vi "PQC_VisualAlignment_contact.vi"() -> ()   [LabVIEW 2020]
uses:
  <vilib>/userdefined/High Color/IMAQdx.ctl
  <vilib>/vision/driver/IMAQdx.llb/IMAQdx Buffer Number Mode.ctl
  <vilib>/Analysis/baseanly.llb/Mean (DBL).vi
  <vilib>/Utility/file.llb/Read Delimited Spreadsheet (string).vi
  <instrlib>/Keithley 700B Series/Keithley 700B Series.lvlib
  <instrlib>/Agilent E4980/Agilent E4980.lvlib
  <vilib>/vision/driver/NI_Vision_Acquisition_Software.lvlib
  <vilib>/Analysis/NI_AALBase.lvlib
panel:
  in  "array 2":dbl[][](array[numeric])=[[999999999.0, 1000000000.0, 1000000000.0, 1000000000.0], [1000000000.0, 1000000000.0, 1000000000.0, 1000000000.0], [1000000000.0, 1000000000.0, 1000000000.0, 1000000000.0], [1000000000.0, 1000000000.0, 1000000000.0, 1000000000.0], [1000000000.0, 1000000000.0, 1000000000.0, 1000000000.0], [1000000000.0, 1000000000.0, 1000000000.0, 1000000000.0], [1000000000.0, 1000000000.0, 1000000000.0, 1000000000.0], [1000000000.0, 1000000000.0, 1000000000.0, 1000000000.0], [1000000000.0, 1000000000.0, 1000000000.0, 1000000000.0], [1000000000.0, 1000000000.0, 1000000000.0, 1000000000.0]] format="%_3e"
  in  "Switch Channel File Path":path=path "C:/Users/Lab User/Desktop/PQC_VisualAlignment/contactSwitchChannels.txt"
  in  "?":enum32{"Data", "Debug and Errors"}(tab)
  out "Rp":dbl[unit]
  out "Cp":dbl[unit]
  in  "Resistance Check":bool
  in  "Measurement Number":i32
  out "Measurement Set":i32
  out "Indicator Cluster":T1
  out "Average of last 3 measurements":dbl[](array[numeric])
  out "Error Out":errorcluster
  in  "stop camera":bool
  in  "Camera ID 2":T2="PQC top"
  out "Frame Rate":dbl
  in  "Start Camera":bool
  in  "Stop Program":bool
  in  "LCR VISA Resource":refnum<visa-resource-name>="GPIB0::19::INSTR"
  in  "707B VISA Resource":refnum<visa-resource-name>="GPIB0::16::INSTR"
  out "PQC Alignment":T3(plugin-control)
  # "2H11, 2B01, 1B01, 2B11, 2B03, 2B04, 2B05, 2B06, 2B07, 2B08, 1H02, 1H03, 1H04, 1H05, 1H06, 1H07, 1H08, 1H09, 2H09, 2H02, 1A11"
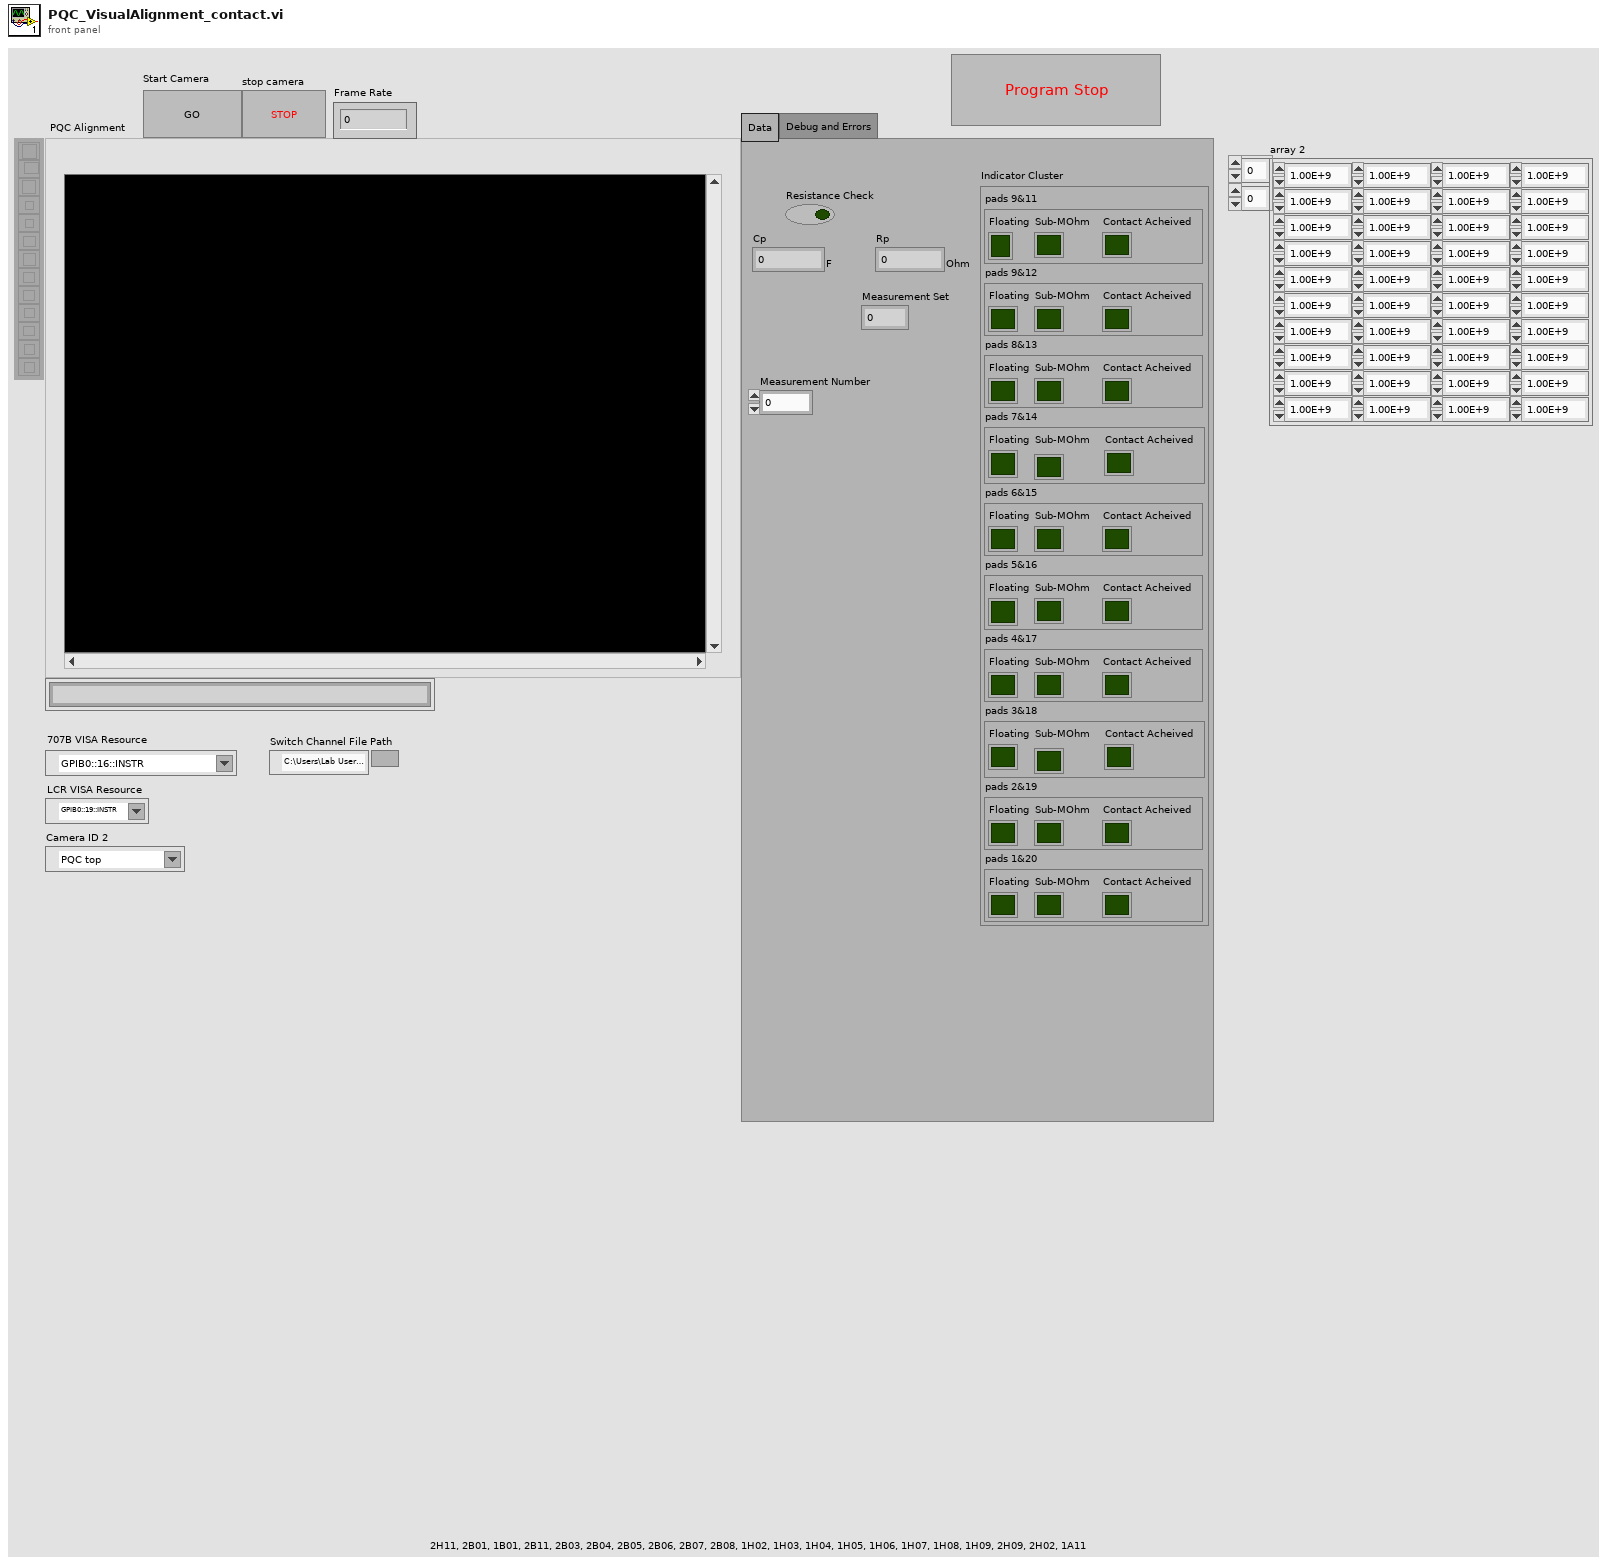
[diagram p1: front panel]
types:
  T1 = cluster{"pads 9&11":cluster{"Floating":bool, "Sub-MOhm":bool, "Contact Acheived":bool}, "pads 9&12":cluster{"Floating":bool, "Sub-MOhm":bool, "Contact Acheived":bool}, "pads 8&13":cluster{"Floating":bool, "Sub-MOhm":bool, "Contact Acheived":bool}, "pads 7&14":cluster{"Floating":bool, "Sub-MOhm":bool, "Contact Acheived":bool}, "pads 6&15":cluster{"Floating":bool, "Sub-MOhm":bool, "Contact Acheived":bool}, "pads 5&16":cluster{"Floating":bool, "Sub-MOhm":bool, "Contact Acheived":bool}, "pads 4&17":cluster{"Floating":bool, "Sub-MOhm":bool, "Contact Acheived":bool}, "pads 3&18":cluster{"Floating":bool, "Sub-MOhm":bool, "Contact Acheived":bool}, "pads 2&19":cluster{"Floating":bool, "Sub-MOhm":bool, "Contact Acheived":bool}, "pads 1&20":cluster{"Floating":bool, "Sub-MOhm":bool, "Contact Acheived":bool}}
  T2 = typedef "IMAQdx.ctl" = refnum<k21>
  T3 = typedef "IMAQ Image.ctl" = refnum<image>
  T4 = cluster{"Floating":bool, "Sub-MOhm":bool, "Contact Acheived":bool}
  T5 = typedef "NI_Vision_Acquisition_Software.lvlib/IMAQdx Buffer Number Mode.ctl" = enum32{"Next", "Last", "Buffer Number", "Every", "Last New"}
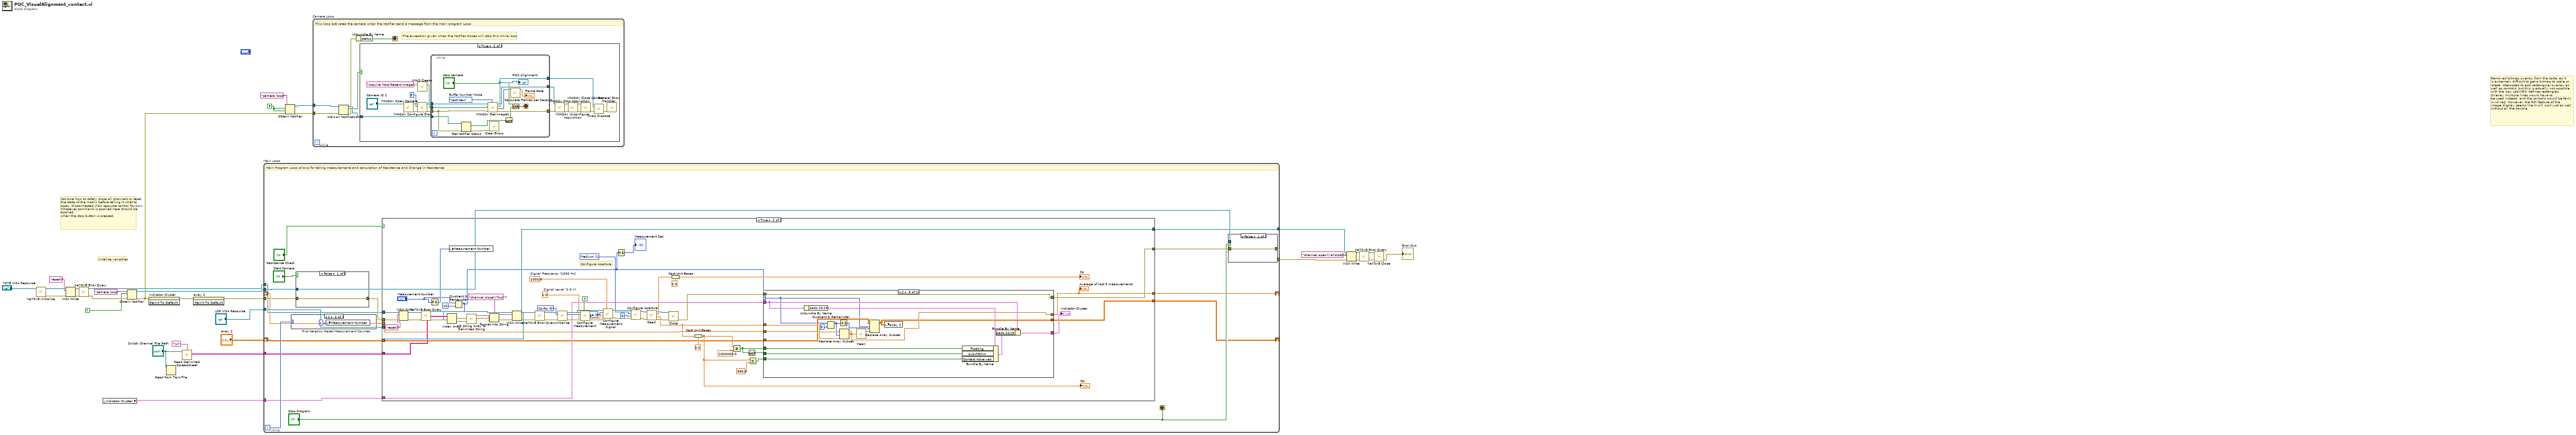
[diagram p0: block diagram]
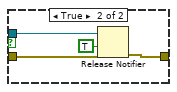
[diagram p3: hidden frame]
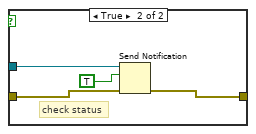
[diagram p5: hidden frame]
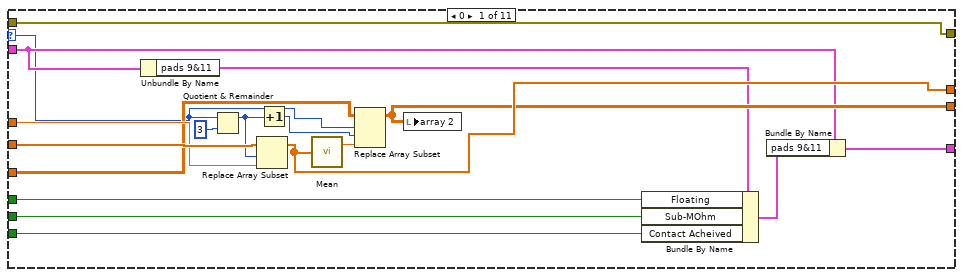
[diagram p7: hidden frame]
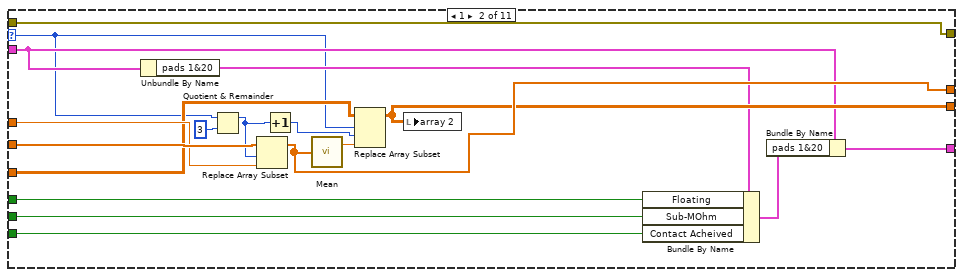
[diagram p8: hidden frame]
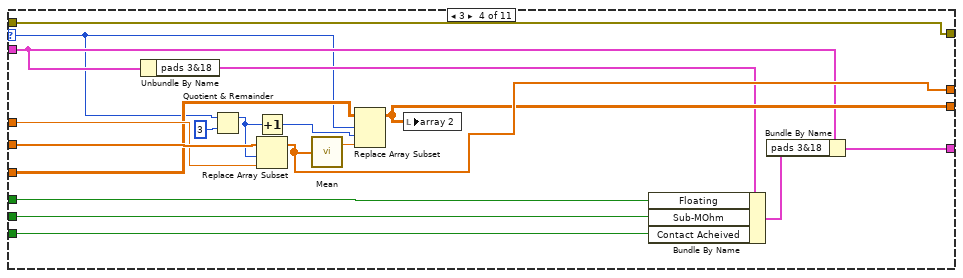
[diagram p9: hidden frame]
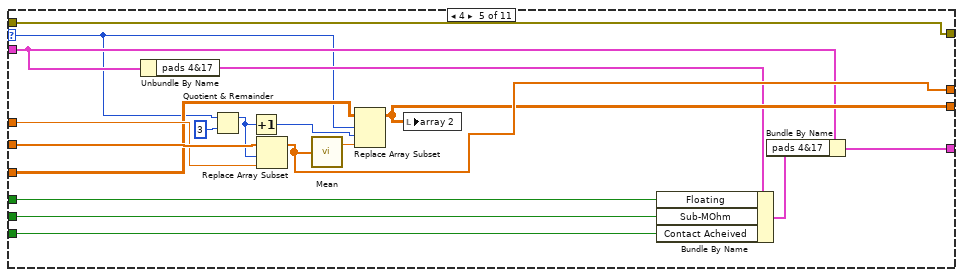
[diagram p10: hidden frame]
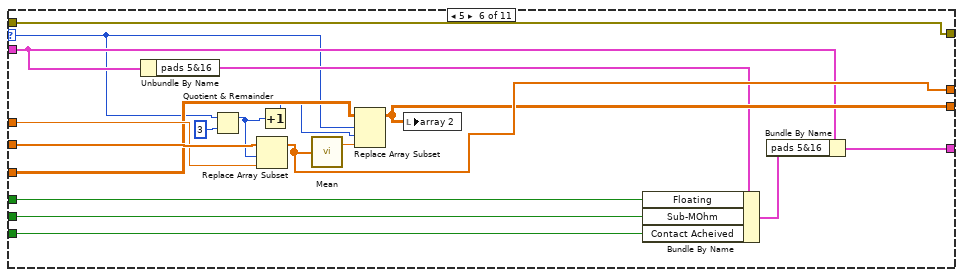
[diagram p11: hidden frame]
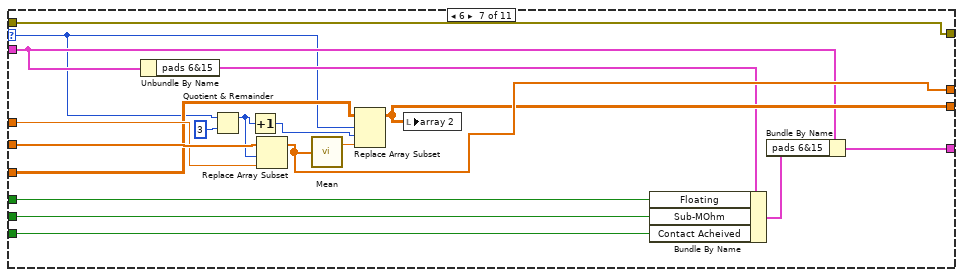
[diagram p12: hidden frame]
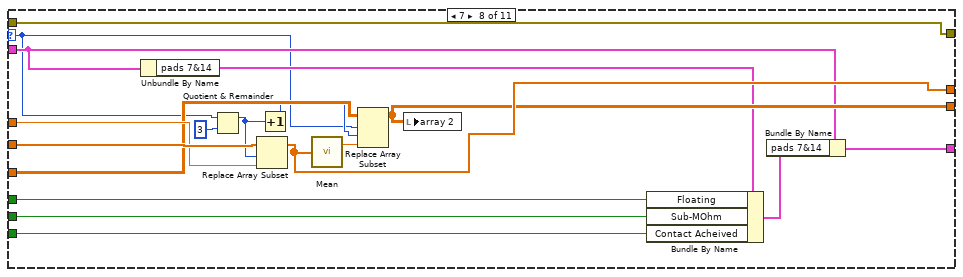
[diagram p13: hidden frame]
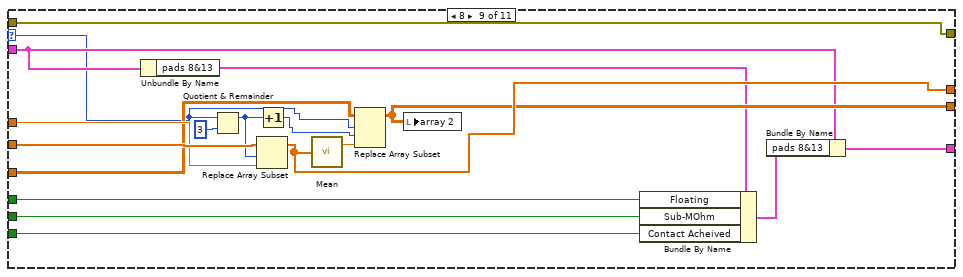
[diagram p14: hidden frame]
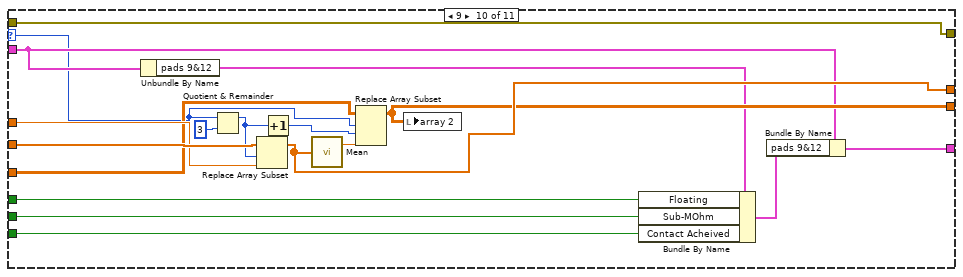
[diagram p15: hidden frame]
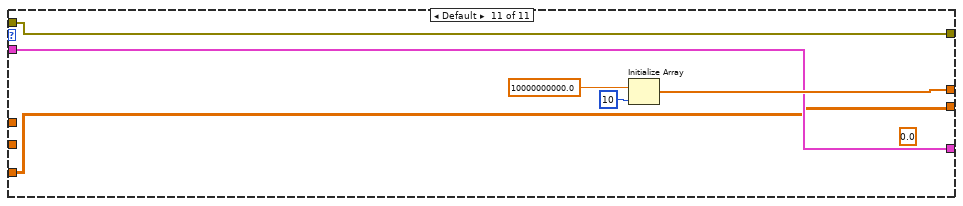
[diagram p16: hidden frame]
diagram:
  w12 = FALSE ("create if not found? (T)")
  # "initalize variables"
  # "Removed bitmap overlay from the code, as it \nis extremely difficult to get a bitmap to scale or\nrotate. Attempted to add rectangular overlay as \nwell as controls, but this is actually not possible \nwith the way LabVIEW defines rectangles. \nOverlay multiple lines would have to \nbe used instead, and the controls would be fairly involved. However, the ROI feature of the \nimage display seems like it will work just as well,\nwithout all the trouble."
  # "Not sure how to safely close all channels or reset the state of the matrix before telling it what to open. Disconnected VISA resource control for now. Whatever command is applied here should be applied\nwhen the stop button is pressed."
  n1 = call <instrlib>:"Ke70xB Initialize.vi"("VISA resource name"="707B VISA Resource") -> ("error out"=w29:errorcluster, "VISA resource name out"=w32:refnum<visa-resource-name>)  [unwired: 9 in]
  n2 = VISA Write(VISA resource name=w32, write buffer="reset()", error in (no error)=w29) -> (VISA resource name out=w30:refnum<visa-resource-name>, error out=w28:errorcluster)  [unwired: 1 out]
  n3 = call <instrlib>:"Ke70xB Error Query.vi"("error in (no error)"=w28, "VISA resource name"=w30) -> ("error out"=w11:errorcluster, "VISA resource name out"=w10:refnum<visa-resource-name>)  [unwired: 6 in, 2 out]
  n4 = local read "Indicator Cluster"() -> (w5:T1)
  n5 = Obtain Notifier(name (unnamed)="camera loop", notification data type=TRUE, error in (no error)=w11) -> (notifier out=w17:refnum<notifier>, error out=w2:errorcluster)  [unwired: 1 in, 1 out]
  n6 = invoke on="Indicator Cluster" class="Clust (strict)" method="Reinit To Default"(error in=w2) -> (error out=w1:errorcluster)  [unwired: 2 in, 2 out]
  n7 = Read from Text File(file (use dialog)="Switch Channel File Path") -> ()  [unwired: 3 in, 4 out]
  n8 = call-poly <vilib>:"Read Delimited Spreadsheet.vi"("file path (dialog if empty)"="Switch Channel File Path", "delimiter (\\t)"="\\n" ("delimiter (\\t)")) -> ("all rows"=w6:string[][])  [unwired: 8 in, 5 out]
  n9 = invoke on="array 2" class="Arr (strict)" method="Reinit To Default"(error in=w1) -> (error out=w4:errorcluster)  [unwired: 2 in, 2 out]
  n10 = while "Main Loop" {
    shift-right: [w44] -> _
    shift-left: _ -> [w45]
    tunnel: w4 -> [w39]
    tunnel: "LCR VISA Resource" -> [w49]
    tunnel: w17 -> [w40]
    tunnel: [w42] -> w16
    tunnel: w10 -> [w38]
    tunnel: [w37] -> w9
    tunnel: w6 -> [w36]
    tunnel: w5 -> [w35]
    shift-right: [w34] -> _
    shift-left: "array 2" -> [w33]
    i -> [w46]
    stop <- "Stop Program" stop-if-true
    # "Main Program Loop allows for taking measurements and calculation of Resistance and Change in Resistance"
    n11 = case "First Iteration Reset Measurement Counter" shown="1" w46 {
      frame 0, Default {
      }
      frame 1 {
        n12 = local write "Measurement Number"(1) -> ()
      }
    }
    n13 = case shown="False" "Start Camera" {
      tunnel: w40 -> [_ w61]
      tunnel: w39 -> [w57 w60]
      tunnel: [w57 w59] -> w47
      frame False {
      }
      frame True {
        # "check status"
        n14 = Send Notification(notification=TRUE, notifier=w61, error in (no error)=w60) -> (error out=w59:errorcluster)  [unwired: 1 out]
      }
    }
    n15 = case shown="True" "Resistance Check" {
      tunnel: w47 -> [w65 w88]
      tunnel: w49 -> [_ w111]
      tunnel: [w65 w102] -> w43
      tunnel: w45 -> [w64 w98]
      tunnel: [w64 w101] -> w44
      tunnel: w38 -> [w63 w85]
      tunnel: [w63 w92] -> w37
      tunnel: w36 -> [_ w83]
      tunnel: w35 -> [_ w78]
      tunnel: [w62 w74] -> w34
      tunnel: w33 -> [w62 w73]
      frame False {
      }
      frame True {
        w117 = u16 1 items=["Short", "Medium", "Long"] ("Measurement Time (1: Medium)")
        w115 = 1.0  # Signal Level (1.0 V)
        w114 = u16 0 items=["Voltage", "Current"] ("Signal Type (0: Voltage)")
        w116 = 1000.0  # Signal Frequency (1000 Hz)
        w112 = u16 3 items=["Cp-D", "Cp-Q", "Cp-G", "Cp-Rp", "Cs-D", "Cs-Q", "Cs-Rs", "Lp-D", "Lp-Q", "Lp-G", "Lp-Rp", "Lp-Rdc", "Ls-D", "Ls-Q", "Ls-Rs", "Ls-Rdc", "R-X", "Z-thd", "Z-thr", "G-B", "Y-thd", "Y-thr", "Vdc-Idc"] ("Function (0: Cp-D)")
        # "Configure Aperture"
        n16 = VISA Write(VISA resource name=w85, write buffer="reset()", error in (no error)=w88) -> (VISA resource name out=w90:refnum<visa-resource-name>, error out=w89:errorcluster)  [unwired: 1 out]
        n17 = call <instrlib>:"Ke70xB Error Query.vi"("error in (no error)"=w89, "VISA resource name"=w90) -> ("error out"=w87:errorcluster, "VISA resource name out"=w86:refnum<visa-resource-name>)  [unwired: 6 in, 2 out]
        n18 = Increment(x="Measurement Number") -> (x+1=w72:i32)
        n19 = local write "Measurement Number"(w72) -> ()
        n20 = Quotient & Remainder(x="Measurement Number", y=10) -> (x-y*floor(x/y)=w70:i32)  [unwired: 1 out]
        n21 = Index Array(array=w83, index (row)=w70) -> (element=w82:string[])  [unwired: 1 in]
        n22 = call <vilib>:"1D String Array to Delimited String.vi"("string array"=w82) -> ("delimited string"=w81:string)  [unwired: 10 in]
        n23 = Format Into String(format string="channel.close(\"%s\")", error in=w87, w81) -> (resulting string=w97:string, error out=w96:errorcluster)  [unwired: 1 in]
        n24 = VISA Write(VISA resource name=w86, write buffer=w97, error in (no error)=w96) -> (VISA resource name out=w93:refnum<visa-resource-name>, error out=w94:errorcluster)  [unwired: 1 out]
        n25 = call <instrlib>:"Ke70xB Error Query.vi"("error in (no error)"=w94, "VISA resource name"=w93) -> ("error out"=w95:errorcluster, "VISA resource name out"=w92:refnum<visa-resource-name>)  [unwired: 6 in, 2 out]
        n26 = call <instrlib>:"Initialize.vi"("error in (no error)"=w95, "VISA resource name"=w111) -> ("error out"=w120:errorcluster, "VISA resource name out"=w119:refnum<visa-resource-name>)  [unwired: 8 in]
        n27 = call <instrlib>:"Configure Measurement.vi"("Enable Auto Range (T:Enable)"=TRUE, "error in (no error)"=w120, "Function (0: Cp-D)"=w112, "VISA resource name"=w119) -> ("error out"=w122:errorcluster, "VISA resource name out"=w121:refnum<visa-resource-name>)  [unwired: 6 in]
        n28 = call <instrlib>:"Configure Measurement Signal.vi"("Signal Frequency (1000 Hz)"=w116, "error in (no error)"=w122, "Signal Level (1.0 V)"=w115, "Signal Type (0: Voltage)"=w114, "VISA resource name"=w121) -> ("error out"=w124:errorcluster, "VISA resource name out"=w123:refnum<visa-resource-name>)  [unwired: 5 in]
        n29 = Increment(x=w70) -> (x+1=→"Measurement Set":i32)
        n30 = call <instrlib>:"Configure Aperture.vi"("error in (no error)"=w124, "Averaging Factor (1)"=0, "Measurement Time (1: Medium)"=w117, "VISA resource name"=w123) -> ("error out"=w107:errorcluster, "VISA resource name out"=w108:refnum<visa-resource-name>)  [unwired: 6 in]
        n31 = call <instrlib>:"Read.vi"("error in (no error)"=w107, "VISA resource name"=w108) -> ("error out"=w110:errorcluster, "Secondary Parameter"=w69:dbl, "Primary Parameter"=w76:dbl, "VISA resource name out"=w109:refnum<visa-resource-name>)  [unwired: 6 in]
        n32 = call <instrlib>:"Close.vi"("error in (no error)"=w110, "VISA resource name"=w109) -> ("error out"=w104:errorcluster)  [unwired: 9 in]
        n33 = Cast Unit Bases(0:w76, 1:dbl[unit] 0.0 ("unit (none)")) -> (2:→"Cp":dbl[unit])
        n34 = Cast Unit Bases(0:w69, 1:dbl[unit] 0.0 ("unit (none)")) -> (2:w67:dbl[unit])
        "Rp" <- w67
        n35 = Greater Or Equal?(x=w67, y=dbl[unit] 1000000.0) -> (x >= y?=w79:bool)
        n36 = Not(x=w79) -> (.not. x?=w80:bool)
        n37 = Less Or Equal?(x=w67, y=dbl[unit] 999.0) -> (x <= y?=w68:bool)
        n38 = case shown="2" w70 {
          selector: w70 -> [w126 w144 w162 w180 w198 w216 w234 w252 w270 w288 _]
          tunnel: [w139 w157 w175 w193 w211 w229 w247 w265 w283 w301 w308] -> w101
          tunnel: w104 -> [w142 w160 w178 w196 w214 w232 w250 w268 w286 w304 w307]
          tunnel: [w142 w160 w178 w196 w214 w232 w250 w268 w286 w304 w307] -> w102
          tunnel: w98 -> [w141 w159 w177 w195 w213 w231 w249 w267 w285 w303 _]
          tunnel: w69 -> [w140 w158 w176 w194 w212 w230 w248 w266 w284 w302 _]
          tunnel: w80 -> [w131 w149 w167 w185 w203 w221 w239 w257 w275 w293 _]
          tunnel: w79 -> [w136 w154 w172 w190 w208 w226 w244 w262 w280 w298 _]
          tunnel: w78 -> [w132 w150 w168 w186 w204 w222 w240 w258 w276 w294 w306]
          tunnel: [w133 w151 w169 w187 w205 w223 w241 w259 w277 w295 w306] -> w77
          tunnel: [w138 w156 w174 w192 w210 w228 w246 w264 w282 w300 w305] -> w74
          tunnel: w73 -> [w137 w155 w173 w191 w209 w227 w245 w263 w281 w299 w305]
          tunnel: w68 -> [w125 w143 w161 w179 w197 w215 w233 w251 w269 w287 _]
          frame 0 {
            n39 = Unbundle By Name(w132) -> ("pads 9&11"=w134:T4)
            n40 = Quotient & Remainder(x=w126, y=i8 3) -> (x-y*floor(x/y)=w128:i32)  [unwired: 1 out]
            n41 = Replace Array Subset(array=w141, new element=w140, index=w128) -> (w139:dbl[])
            n42 = Increment(x=w128) -> (x+1=w127:i32)
            n43 = call-poly <vilib>:"Mean.vi"("X"=w139) -> ("mean"=w129:dbl)  [unwired: 1 out]
            n44 = Replace Array Subset(array=w137, new element=w129, index (row)=w126, index (col)=w127) -> (w138:dbl[][])
            n45 = local write "array 2"(w138) -> ()
            n46 = Bundle By Name(cluster=w134, "Floating"=w136, "Sub-MOhm"=w131, "Contact Acheived"=w125) -> (w135:T4)
            n47 = Bundle By Name(cluster=w132, "pads 9&11"=w135) -> (w133:T1)
          }
          frame 1 {
            n48 = Unbundle By Name(w150) -> ("pads 1&20"=w152:T4)
            n49 = Quotient & Remainder(x=w144, y=i8 3) -> (x-y*floor(x/y)=w146:i32)  [unwired: 1 out]
            n50 = Replace Array Subset(array=w159, new element=w158, index=w146) -> (w157:dbl[])
            n51 = Increment(x=w146) -> (x+1=w145:i32)
            n52 = call-poly <vilib>:"Mean.vi"("X"=w157) -> ("mean"=w147:dbl)  [unwired: 1 out]
            n53 = Replace Array Subset(array=w155, new element=w147, index (row)=w144, index (col)=w145) -> (w156:dbl[][])
            n54 = local write "array 2"(w156) -> ()
            n55 = Bundle By Name(cluster=w152, "Floating"=w154, "Sub-MOhm"=w149, "Contact Acheived"=w143) -> (w153:T4)
            n56 = Bundle By Name(cluster=w150, "pads 1&20"=w153) -> (w151:T1)
          }
          frame 2 {
            n57 = Unbundle By Name(w168) -> ("pads 2&19"=w170:T4)
            n58 = Quotient & Remainder(x=w162, y=i8 3) -> (x-y*floor(x/y)=w164:i32)  [unwired: 1 out]
            n59 = Increment(x=w164) -> (x+1=w163:i32)
            n60 = Replace Array Subset(array=w177, new element=w176, index=w164) -> (w175:dbl[])
            n61 = call-poly <vilib>:"Mean.vi"("X"=w175) -> ("mean"=w165:dbl)  [unwired: 1 out]
            n62 = Replace Array Subset(array=w173, new element=w165, index (row)=w162, index (col)=w163) -> (w174:dbl[][])
            n63 = local write "array 2"(w174) -> ()
            n64 = Bundle By Name(cluster=w170, "Floating"=w172, "Sub-MOhm"=w167, "Contact Acheived"=w161) -> (w171:T4)
            n65 = Bundle By Name(cluster=w168, "pads 2&19"=w171) -> (w169:T1)
          }
          frame 3 {
            n66 = Unbundle By Name(w186) -> ("pads 3&18"=w188:T4)
            n67 = Quotient & Remainder(x=w180, y=i8 3) -> (x-y*floor(x/y)=w182:i32)  [unwired: 1 out]
            n68 = Increment(x=w182) -> (x+1=w181:i32)
            n69 = Replace Array Subset(array=w195, new element=w194, index=w182) -> (w193:dbl[])
            n70 = call-poly <vilib>:"Mean.vi"("X"=w193) -> ("mean"=w183:dbl)  [unwired: 1 out]
            n71 = Replace Array Subset(array=w191, new element=w183, index (row)=w180, index (col)=w181) -> (w192:dbl[][])
            n72 = local write "array 2"(w192) -> ()
            n73 = Bundle By Name(cluster=w188, "Floating"=w190, "Sub-MOhm"=w185, "Contact Acheived"=w179) -> (w189:T4)
            n74 = Bundle By Name(cluster=w186, "pads 3&18"=w189) -> (w187:T1)
          }
          frame 4 {
            n75 = Unbundle By Name(w204) -> ("pads 4&17"=w206:T4)
            n76 = Quotient & Remainder(x=w198, y=i8 3) -> (x-y*floor(x/y)=w200:i32)  [unwired: 1 out]
            n77 = Increment(x=w200) -> (x+1=w199:i32)
            n78 = Replace Array Subset(array=w213, new element=w212, index=w200) -> (w211:dbl[])
            n79 = call-poly <vilib>:"Mean.vi"("X"=w211) -> ("mean"=w201:dbl)  [unwired: 1 out]
            n80 = Replace Array Subset(array=w209, new element=w201, index (row)=w198, index (col)=w199) -> (w210:dbl[][])
            n81 = local write "array 2"(w210) -> ()
            n82 = Bundle By Name(cluster=w206, "Floating"=w208, "Sub-MOhm"=w203, "Contact Acheived"=w197) -> (w207:T4)
            n83 = Bundle By Name(cluster=w204, "pads 4&17"=w207) -> (w205:T1)
          }
          frame 5 {
            n84 = Unbundle By Name(w222) -> ("pads 5&16"=w224:T4)
            n85 = Quotient & Remainder(x=w216, y=i8 3) -> (x-y*floor(x/y)=w218:i32)  [unwired: 1 out]
            n86 = Replace Array Subset(array=w231, new element=w230, index=w218) -> (w229:dbl[])
            n87 = Increment(x=w218) -> (x+1=w217:i32)
            n88 = call-poly <vilib>:"Mean.vi"("X"=w229) -> ("mean"=w219:dbl)  [unwired: 1 out]
            n89 = Replace Array Subset(array=w227, new element=w219, index (row)=w216, index (col)=w217) -> (w228:dbl[][])
            n90 = local write "array 2"(w228) -> ()
            n91 = Bundle By Name(cluster=w224, "Floating"=w226, "Sub-MOhm"=w221, "Contact Acheived"=w215) -> (w225:T4)
            n92 = Bundle By Name(cluster=w222, "pads 5&16"=w225) -> (w223:T1)
          }
          frame 6 {
            n93 = Unbundle By Name(w240) -> ("pads 6&15"=w242:T4)
            n94 = Quotient & Remainder(x=w234, y=i8 3) -> (x-y*floor(x/y)=w235:i32)  [unwired: 1 out]
            n95 = Increment(x=w235) -> (x+1=w236:i32)
            n96 = Replace Array Subset(array=w249, new element=w248, index=w235) -> (w247:dbl[])
            n97 = call-poly <vilib>:"Mean.vi"("X"=w247) -> ("mean"=w237:dbl)  [unwired: 1 out]
            n98 = Replace Array Subset(array=w245, new element=w237, index (row)=w234, index (col)=w236) -> (w246:dbl[][])
            n99 = local write "array 2"(w246) -> ()
            n100 = Bundle By Name(cluster=w242, "Floating"=w244, "Sub-MOhm"=w239, "Contact Acheived"=w233) -> (w243:T4)
            n101 = Bundle By Name(cluster=w240, "pads 6&15"=w243) -> (w241:T1)
          }
          frame 7 {
            n102 = Unbundle By Name(w258) -> ("pads 7&14"=w260:T4)
            n103 = Quotient & Remainder(x=w252, y=i8 3) -> (x-y*floor(x/y)=w254:i32)  [unwired: 1 out]
            n104 = Replace Array Subset(array=w267, new element=w266, index=w254) -> (w265:dbl[])
            n105 = Increment(x=w254) -> (x+1=w253:i32)
            n106 = call-poly <vilib>:"Mean.vi"("X"=w265) -> ("mean"=w255:dbl)  [unwired: 1 out]
            n107 = Replace Array Subset(array=w263, new element=w255, index (row)=w252, index (col)=w253) -> (w264:dbl[][])
            n108 = local write "array 2"(w264) -> ()
            n109 = Bundle By Name(cluster=w260, "Floating"=w262, "Sub-MOhm"=w257, "Contact Acheived"=w251) -> (w261:T4)
            n110 = Bundle By Name(cluster=w258, "pads 7&14"=w261) -> (w259:T1)
          }
          frame 8 {
            n111 = Unbundle By Name(w276) -> ("pads 8&13"=w278:T4)
            n112 = Quotient & Remainder(x=w270, y=i8 3) -> (x-y*floor(x/y)=w272:i32)  [unwired: 1 out]
            n113 = Replace Array Subset(array=w285, new element=w284, index=w272) -> (w283:dbl[])
            n114 = Increment(x=w272) -> (x+1=w271:i32)
            n115 = call-poly <vilib>:"Mean.vi"("X"=w283) -> ("mean"=w273:dbl)  [unwired: 1 out]
            n116 = Replace Array Subset(array=w281, new element=w273, index (row)=w270, index (col)=w271) -> (w282:dbl[][])
            n117 = local write "array 2"(w282) -> ()
            n118 = Bundle By Name(cluster=w278, "Floating"=w280, "Sub-MOhm"=w275, "Contact Acheived"=w269) -> (w279:T4)
            n119 = Bundle By Name(cluster=w276, "pads 8&13"=w279) -> (w277:T1)
          }
          frame 9 {
            n120 = Unbundle By Name(w294) -> ("pads 9&12"=w296:T4)
            n121 = Quotient & Remainder(x=w288, y=i8 3) -> (x-y*floor(x/y)=w290:i32)  [unwired: 1 out]
            n122 = Replace Array Subset(array=w303, new element=w302, index=w290) -> (w301:dbl[])
            n123 = Increment(x=w290) -> (x+1=w289:i32)
            n124 = call-poly <vilib>:"Mean.vi"("X"=w301) -> ("mean"=w291:dbl)  [unwired: 1 out]
            n125 = Replace Array Subset(array=w299, new element=w291, index (row)=w288, index (col)=w289) -> (w300:dbl[][])
            n126 = local write "array 2"(w300) -> ()
            n127 = Bundle By Name(cluster=w296, "Floating"=w298, "Sub-MOhm"=w293, "Contact Acheived"=w287) -> (w297:T4)
            n128 = Bundle By Name(cluster=w294, "pads 9&12"=w297) -> (w295:T1)
          }
          frame Default {
            (unwired) 0.0
            n129 = Initialize Array(10000000000.0 ("element"), 10 ("dimension size")) -> (w308:dbl[])
          }
        }
        "Average of last 3 measurements" <- w101
        "Indicator Cluster" <- w77
      }
    }
    n130 = case shown="False" "Stop Program" {
      tunnel: w40 -> [_ w53]
      tunnel: w43 -> [w51 w52]
      tunnel: [w51 w55] -> w42
      frame False {
      }
      frame True {
        n131 = Release Notifier(notifier=w53, force destroy? (F)=TRUE, error in (no error)=w52) -> (error out=w55:errorcluster)  [unwired: 2 out]
      }
    }
  }
  n132 = Obtain Notifier(name (unnamed)="camera loop", notification data type=w12, create if not found? (T)=w12, error in (no error)=w2) -> (notifier out=w15:refnum<notifier>, error out=w14:errorcluster)  [unwired: 1 out]
  n133 = while "Camera Loop" {
    tunnel: w15 -> [w312]
    tunnel: w14 -> [w311]
    stop <- w314 stop-if-true
    # "The exception given when the Notifier closes will stop this while loop"
    # "This loop activates the camera when the Notifier send a message from the main program Loop"
    n134 = Wait on Notification(notifier=w312, error in (no error)=w311) -> (notifier out=w313:refnum<notifier>, notification=w316:bool, error out=w315:errorcluster)  [unwired: 2 in, 1 out]
    n135 = Unbundle By Name(w315) -> ("status"=w314:bool)
    n136 = case shown="True" w316 {
      tunnel: w313 -> [_ w317]
      frame False {
      }
      frame True {
        n137 = call <vilib>:"IMAQdx Open Camera.vi"("Session In"="Camera ID 2") -> ("error out"=w318:errorcluster, "Session Out"=w323:T2)  [unwired: 2 in, 7 out]
        n138 = call "IMAQ Create"("Image Name"="Acquire Most Recent Image") -> ("New Image"=w334:T3)  [unwired: 3 in, 2 out]
        n139 = call <vilib>:"IMAQdx Configure Grab.vi"("error in"=w318, "Number of Buffers"=u32 5, "Session In"=w323) -> ("error out"=w321:errorcluster, "Session Out"=w322:T2)  [unwired: 7 in]
        n140 = while {
          tunnel: [w346] -> w332
          tunnel: w321 -> [w336]
          tunnel: w322 -> [w349]
          tunnel: [w339] -> w333
          tunnel: w334 -> [w348]
          tunnel: [w343] -> w324
          tunnel: w317 -> [w342]
          stop <- w340 stop-if-true
          w347 = IMAQdx_Buffer_Number_Mode."Last New"  # Buffer Number Mode
          n141 = Get Notifier Status(notifier=w342, error in (no error)=w336) -> (current notification=w337:bool, error out=w335:errorcluster)  [unwired: 3 out]
          n142 = call <vilib>:"IMAQdx Get Image2.vi"("Buffer Number Mode (Next)"=w347, "error in"=w336, "Image In"=w348, "Session In"=w349) -> ("error out"=w339:errorcluster, "Buffer Number Out"=w345:u32, "Image Out"=w343:T3, "Session Out"=w346:T2)  [unwired: 4 in]
          "PQC Alignment" <- w343
          n143 = call <vilib>:"Clear Errors.vi"("error in (no error)"=w335) -> ()  [unwired: 5 in, 2 out]
          n144 = Not(x=w337) -> (.not. x?=w338:bool)
          n145 = call <vilib>:"Calculate Frames per Second.vi"("Buffer Number"=w345) -> ("Acquired Frames/s"=→"Frame Rate":dbl)  [unwired: 8 in, 2 out]
          n146 = Or(x="stop camera", y=w338) -> (x .or. y?=w340:bool)
        }
        n147 = call <vilib>:"IMAQdx Stop Acquisition.vi"("error in"=w333, "Session In"=w332) -> ("error out"=w328:errorcluster, "Session Out"=w329:T2)  [unwired: 8 out]
        n148 = call <vilib>:"IMAQdx Unconfigure Acquisition.vi"("error in"=w328, "Session In"=w329) -> ("error out"=w331:errorcluster, "Session Out"=w330:T2)  [unwired: 8 out]
        n149 = call <vilib>:"IMAQdx Close Camera.vi"("error in"=w331, "Session In"=w330) -> ("error out"=w327:errorcluster)  [unwired: 9 out]
        n150 = call "Imaq Dispose"("Image"=w324, "error in (no error)"=w327) -> ("error out"=w326:errorcluster)  [unwired: 4 in]
        n151 = call <vilib>:"General Error Handler.vi"("error in (no error)"=w326) -> ()  [unwired: 2 in, 13 out]
      }
    }
  }
  n152 = VISA Write(VISA resource name=w9, write buffer="channel.open(\"allslots\")", error in (no error)=w16) -> (VISA resource name out=w22:refnum<visa-resource-name>, error out=w18:errorcluster)  [unwired: 1 out]
  n153 = call <instrlib>:"Ke70xB Error Query.vi"("error in (no error)"=w18, "VISA resource name"=w22) -> ("error out"=w20:errorcluster, "VISA resource name out"=w19:refnum<visa-resource-name>)  [unwired: 6 in, 2 out]
  n154 = call <instrlib>:"Ke70xB Close.vi"("error in (no error)"=w20, "VISA resource name"=w19) -> ("error out"=→"Error Out":errorcluster)  [unwired: 9 in]
